vi "LV2 for Class Objects.vi"(6 "Command":enum16{"Get", "Set"}(ring), 11 "Variant In":variant) -> (3 "Variant Out":variant)   [LabVIEW 2016, in "SLL Class.lvlib"]
doc: "LV2 Global for Variant LUT, which stores the class objects."
uses:
  SLL Class.lvlib
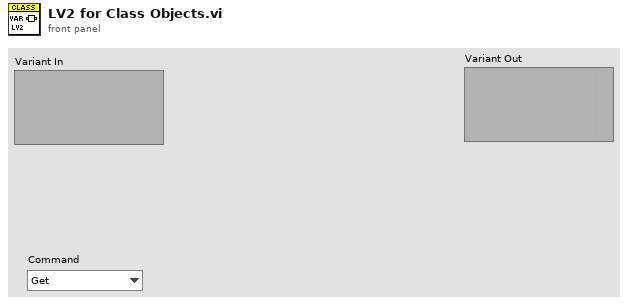
[diagram p1: front panel]
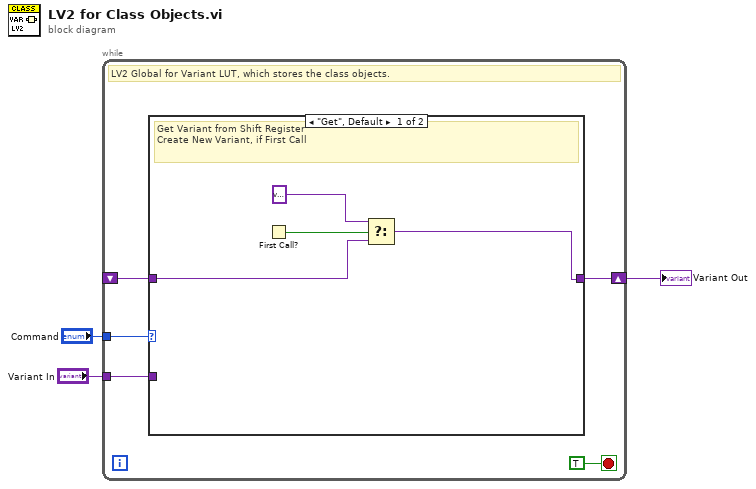
[diagram p0: block diagram]
diagram:
  n1 = while {
    shift-right: [w6] -> w2
    shift-left: _ -> [w4]
    tunnel: "Command" -> [w7]
    tunnel: "Variant In" -> [w5]
    stop <- TRUE stop-if-true
    # "LV2 Global for Variant LUT, which stores the class objects."
    n2 = case shown="\"Get\", Default" w7 {
      tunnel: [w9 w13] -> w6
      tunnel: w5 -> [_ w13]
      tunnel: w4 -> [w10 _]
      frame "Get", Default {
        # "Get Variant from Shift Register\nCreate New Variant, if First Call"
        n3 = First Call?() -> (First Call?: T/F=w11:bool)
        n4 = Select(t=variant, s=w11, f=w10) -> (s? t:f=w9:variant)
      }
      frame "Set" {
      }
    }
  }
  "Variant Out" <- w2
